vi "Motic Set ROI.vi"(0 "camera":i32, 1 "top":i32, 2 "left":i32, 3 "bottom":i32, 4 "right":i32, 5 "error in (no error)":errorcluster) -> (14 "camera out":i32, 15 "matrix top out":i32, 16 "matrix left out":i32, 17 "matrix bottom out":i32, 18 "matrix bottom out":i32, 19 "error out":errorcluster)   [LabVIEW 2012, in "MoticApi.lvlib"]
doc: "MOTICAPI bool Motic_SetROI(MUCam_Handle camera, int *top, int *left, int *bottom, int *right);"
uses:
  MoticApi.lvlib
  MoticApi.dll
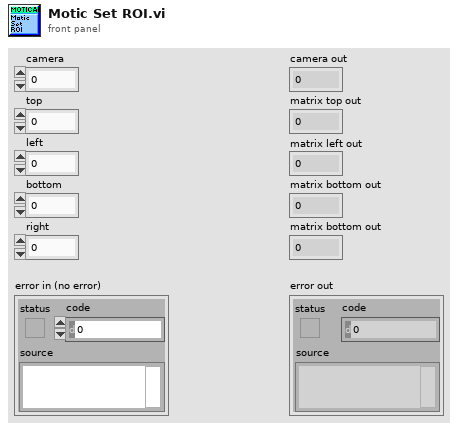
[diagram p1: front panel]
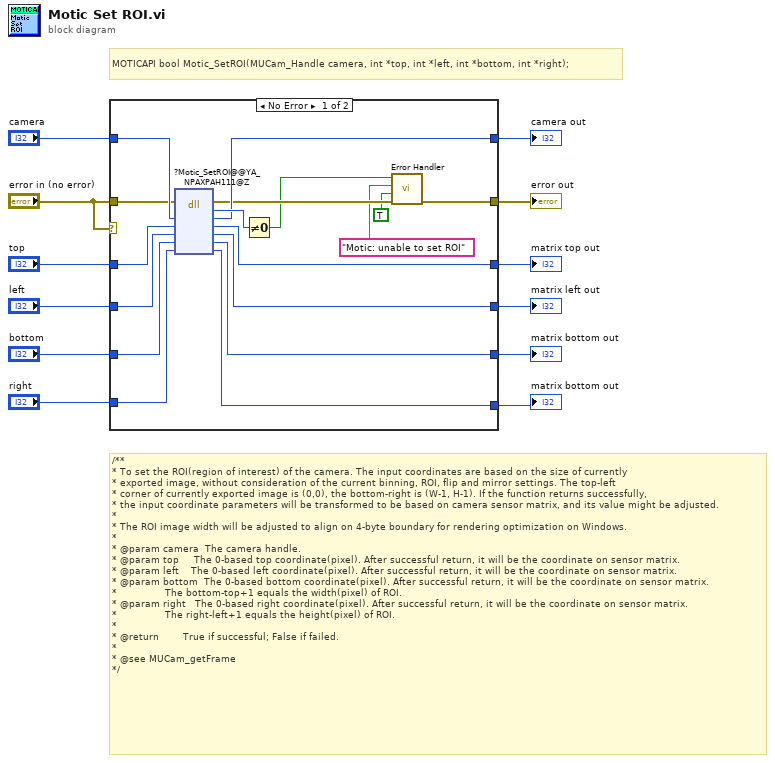
[diagram p0: block diagram]
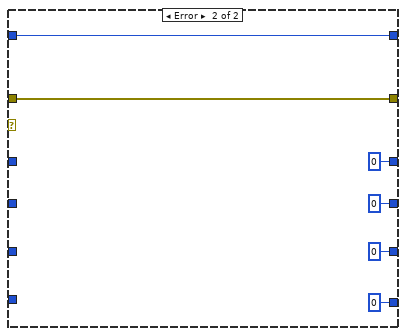
[diagram p2: hidden frame]
diagram:
  # "/**\n* To set the ROI(region of interest) of the camera. The input coordinates are based on the size of currently\n* exported image, without consideration of the current binning, ROI, flip and mirror settings. The top-left\n* corner of currently exported image is (0,0), the bottom-right is (W-1, H-1). If the function returns successfully,\n* the input coordinate parameters will be transformed to be based on camera sensor matrix, and its value might be adjusted.\n*\n* The ROI image width will be adjusted to align on 4-byte boundary for rendering optimization on Windows.\n*\n* @param camera  The camera handle.\n* @param top     The 0-based top coordinate(pixel). After successful return, it will be the coordinate on sensor matrix.\n* @param left    The 0-based left coordinate(pixel). After successful return, it will be the coordinate on sensor matrix.\n* @param bottom  The 0-based bottom coordinate(pixel). After successful return, it will be the coordinate on sensor matrix.\n*                The bottom-top+1 equals the width(pixel) of ROI.\n* @param right   The 0-based right coordinate(pixel). After successful return, it will be the coordinate on sensor matrix.\n*                The right-left+1 equals the height(pixel) of ROI.\n*\n* @return        True if successful; False if failed.\n*\n* @see MUCam_getFrame\n*/"
  # "MOTICAPI bool Motic_SetROI(MUCam_Handle camera, int *top, int *left, int *bottom, int *right);"
  n1 = case shown="No Error" "error in (no error)" {
    tunnel: "camera" -> [w28 w34]
    tunnel: [w27 w34] -> w11
    tunnel: "top" -> [w26 _]
    tunnel: "left" -> [w25 _]
    tunnel: "bottom" -> [w24 _]
    tunnel: "right" -> [w23 _]
    tunnel: [w18 w35] -> w6
    tunnel: "error in (no error)" -> [w17 w35]
    tunnel: [w16 0 ("top")] -> w5
    tunnel: [w15 0 ("left")] -> w4
    tunnel: [w14 0 ("bottom")] -> w3
    tunnel: [w13 0 ("right")] -> w2
    frame No Error {
      n2 = dll-call lib="C:/Users/TTS-Digital/Desktop/MoticApi/MoticApi_git/MoticApi/MoticApi.*" fn="?Motic_SetROI@@YA_NPAXPAH111@Z"(error in=w17, "camera"=w28, "top"=w26, "left"=w25, "bottom"=w24, "right"=w23) -> (error out=w22:errorcluster, "return type"=w29:u8, "camera"=w27:i32, "top"=w16:i32, "left"=w15:i32, "bottom"=w14:i32, "right"=w13:i32)  [unwired: 2 in, 1 out]
      n3 = Not Equal To 0?(x=w29) -> (x != 0?=w21:bool)
      n4 = call "Error Handler.vi"("error in (no error)"=w22, "Is warning?"=TRUE, "Error message"="Motic: unable to set ROI", "Function return"=w21) -> ("error out"=w18:errorcluster)  [unwired: 7 in]
    }
    frame Error {
    }
  }
  "camera out" <- w11
  "error out" <- w6
  "matrix top out" <- w5
  "matrix left out" <- w4
  "matrix bottom out" <- w3
  "matrix bottom out" <- w2
